vi "Send Motor Command.vi"(7 "Timestep (s)":dbl, 8 "error in (no error)":errorcluster, 9 "Turning Radius":dbl, 10 "Speed (units/s)":dbl, 11 "Simulator in":refnum<class "Simulator.lvclass">) -> (0 "error out":errorcluster, 1 "Bearing Out":dbl, 2 "Pose Out":cluster{dbl, dbl}, 3 "Simulator out":refnum<class "Simulator.lvclass">)   [LabVIEW 2011, in "Simulator.lvclass"]
uses:
  Simulator.lvclass
  Simulator.lvclass/Simulator.ctl
  <vilib>/Analysis/baseanly.llb/A x Vector.vi
  <vilib>/Analysis/NI_AALBase.lvlib
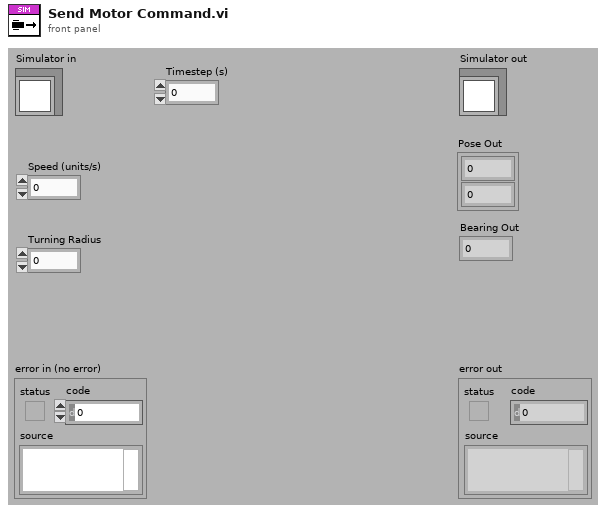
[diagram p1: front panel]
types:
  T1 = typedef "NI_Matrix.lvlib/RealMatrix.ctl" = dbl[][]
  T2 = cluster{"A x Vector[0]":dbl, "A x Vector[1]":dbl}
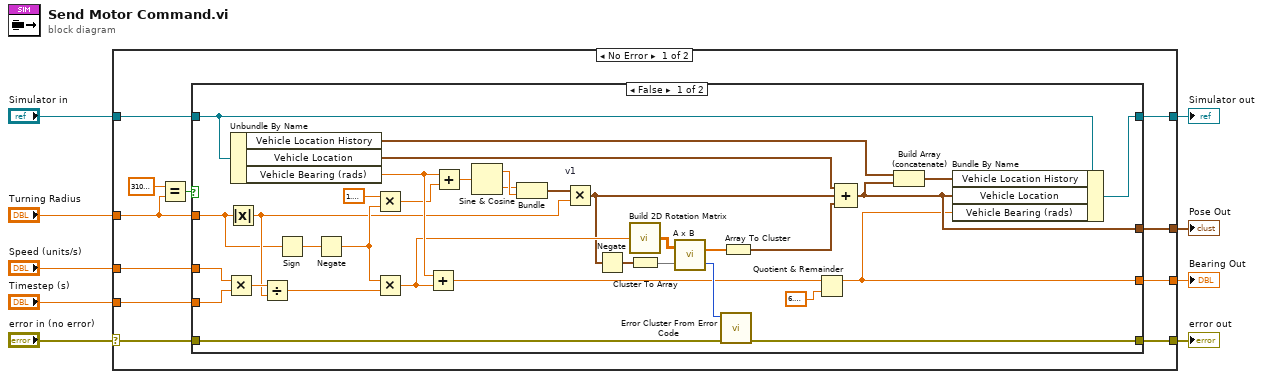
[diagram p0: block diagram]
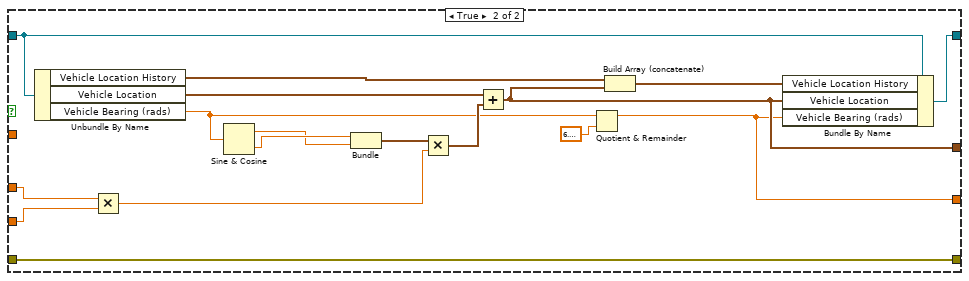
[diagram p2: hidden frame]
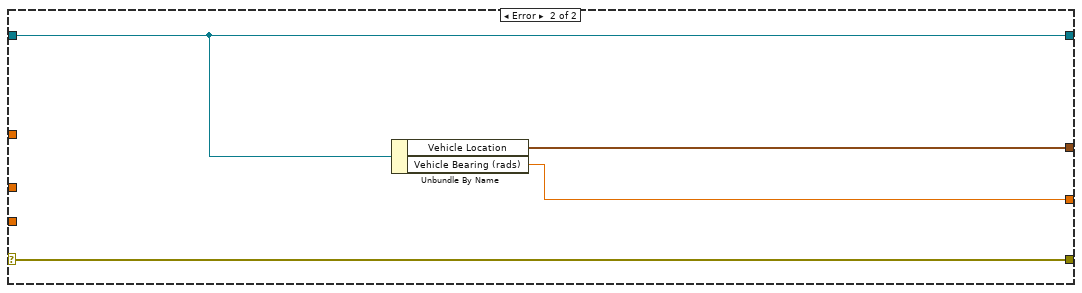
[diagram p3: hidden frame]
diagram:
  n1 = case shown="No Error" "error in (no error)" {
    selector: "error in (no error)" -> [w14 w75]
    tunnel: [w13 w75] -> w8
    tunnel: [w17 w74] -> w6
    tunnel: "Simulator in" -> [w18 w74]
    tunnel: "Speed (units/s)" -> [w20 _]
    tunnel: "Turning Radius" -> [w10 _]
    tunnel: "Timestep (s)" -> [w19 _]
    tunnel: [w16 w72] -> w2
    tunnel: [w15 w73] -> w1
    frame No Error {
      n2 = Equal?(x=31000000000.0, y=w10) -> (x = y?=w12:bool)
      n3 = case shown="False" w12 {
        tunnel: w20 -> [w53 w62]
        tunnel: w19 -> [w52 w61]
        tunnel: w18 -> [w48 w71]
        tunnel: [w47 w70] -> w17
        tunnel: [w43 w57] -> w16
        tunnel: [w21 w56] -> w15
        tunnel: w14 -> [w40 w69]
        tunnel: [w39 w69] -> w13
        tunnel: w10 -> [w26 _]
        frame False {
          n4 = Multiply(x=w53, y=w52) -> (x*y=w54:dbl)
          n5 = Absolute Value(x=w26) -> (abs(x)=w27:dbl)
          n6 = Unbundle By Name(w48) -> ("Vehicle Location History"=w45:cluster{"x":dbl, "y":dbl}[], "Vehicle Location"=w44:cluster{"x":dbl, "y":dbl}, "Vehicle Bearing (rads)"=w49:dbl)
          n7 = Divide(x=w54, y=w27) -> (x/y=w32:dbl)
          n8 = Sign(1:w26) -> (0:w31:dbl)
          n9 = Negate(x=w31) -> (-x=w28:dbl)
          n10 = Multiply(x=1.5707963267948966, y=w28) -> (x*y=w30:dbl)
          n11 = Multiply(x=w28, y=w32) -> (x*y=w25:dbl)
          n12 = Add(x=w49, y=w25) -> (x+y=w22:dbl)
          n13 = Add(x=w49, y=w30) -> (x+y=w33:dbl)
          n14 = Sine & Cosine(0:w33) -> (1:w51:dbl, 2:w50:dbl)
          n15 = Bundle(w50, w51) -> (w36:cluster{dbl, dbl})  [unwired: 1 in]
          n16 = Multiply "v1"(x=w36, y=w27) -> (x*y=w24:cluster{dbl, dbl})
          n17 = Negate(x=w24) -> (-x=w35:cluster{dbl, dbl})
          n18 = call "Build 2D Rotation Matrix.vi"("Rotation Angle (rads)"=w25) -> ("Rotation Matrix"=w42:T1)
          n19 = Cluster To Array(cluster=w35) -> (array=w38:dbl[])
          n20 = call-poly <vilib>:"A x B.vi"("Vector"=w38, "A"=w42) -> ("error"=w41:i32, "A x Vector"=w37:dbl[])
          n21 = call <vilib>:"Error Cluster From Error Code.vi"("error in (no error)"=w40, "error code (0)"=w41) -> ("error out"=w39:errorcluster)  [unwired: 7 in]
          n22 = Array To Cluster(array=w37) -> (cluster=w34:T2)
          n23 = Quotient & Remainder(x=w22, y=6.283185307179586) -> (x-y*floor(x/y)=w21:dbl)  [unwired: 1 out]
          n24 = Compound Arithmetic op=ADD(w44, w24, w34) -> (w43:cluster{dbl, dbl})
          n25 = Build Array (concatenate)(w45, w43) -> (w46:cluster{"x":dbl, "y":dbl}[])
          n26 = Bundle By Name(cluster=w48, "Vehicle Location History"=w46, "Vehicle Location"=w43, "Vehicle Bearing (rads)"=w21) -> (w47:refnum<class "Simulator.lvclass">)
        }
        frame True {
          n27 = Unbundle By Name(w71) -> ("Vehicle Location History"=w67:cluster{"x":dbl, "y":dbl}[], "Vehicle Location"=w64:cluster{"x":dbl, "y":dbl}, "Vehicle Bearing (rads)"=w63:dbl)
          n28 = Multiply(x=w62, y=w61) -> (x*y=w60:dbl)
          n29 = Sine & Cosine(0:w63) -> (1:w58:dbl, 2:w59:dbl)
          n30 = Bundle(w59, w58) -> (w66:cluster{dbl, dbl})  [unwired: 1 in]
          n31 = Multiply(x=w66, y=w60) -> (x*y=w65:cluster{dbl, dbl})
          n32 = Add(x=w64, y=w65) -> (x+y=w57:cluster{dbl, dbl})
          n33 = Quotient & Remainder(x=w63, y=6.283185307179586) -> (x-y*floor(x/y)=w56:dbl)  [unwired: 1 out]
          n34 = Build Array (concatenate)(w67, w57) -> (w68:cluster{"x":dbl, "y":dbl}[])
          n35 = Bundle By Name(cluster=w71, "Vehicle Location History"=w68, "Vehicle Location"=w57, "Vehicle Bearing (rads)"=w56) -> (w70:refnum<class "Simulator.lvclass">)
        }
      }
    }
    frame Error {
      n36 = Unbundle By Name(w74) -> ("Vehicle Location"=w72:cluster{"x":dbl, "y":dbl}, "Vehicle Bearing (rads)"=w73:dbl)
    }
  }
  "error out" <- w8
  "Simulator out" <- w6
  "Pose Out" <- w2
  "Bearing Out" <- w1
